vi "UniPend - ControlDesign.vi"() -> ()   [LabVIEW 2012]
uses:
  <vilib>/addons/Control Design/_Model Construction/Model Typedefs.llb/CD State Space Model (MIMO).ctl
  <vilib>/addons/Control Design/_Model Construction/Model Typedefs.llb/CD General Elements.ctl
  <vilib>/addons/Control Design/_Utility/Model Viewer.llb/Model Viewer SubVI/cd_Draw State-Space Equation (SS).vi
  <vilib>/addons/Control Design/_State Feedback Control/State Feedback Control.llb/State Feedback Control SubVis/cd_Discretized Linear Quadratic Regulator.vi
  <vilib>/addons/Control Design/_Model Conversions/Continuous and Discrete.llb/Continuous and Discrete SubVI/cd_Convert Continuous to Discrete (SS).vi
  <vilib>/addons/Control Design/_State Feedback Control/State Feedback Control.llb/CD State Regulator.vi
  <vilib>/addons/Control Design/_Model Reduction/Model Reduction.llb/Model Reduction SubVIs/cd_Remove I-O-S from SS Model.vi
  <vilib>/addons/Control Design/_Frequency Response Analysis/Frequency Response.llb/Frequency Response subVI/cd_Bode (State Space).vi
  <vilib>/addons/Control Design/_Time Response Analysis/Time Response.llb/Time Response subVI/cd_Impulse Response (State-Space).vi
  <vilib>/addons/Control Design/_Time Response Analysis/Time Response.llb/Time Response subVI/cd_Parametric Time Response (SS with External Response).vi
  <vilib>/addons/Control Design/_Dynamic Analysis/Dynamic Analysis.llb/Dynamic Analysis subVI/cd_Pole-Zero Map (State-Space).vi
  <vilib>/addons/Control Design/_Dynamic Analysis/Dynamic Analysis.llb/Dynamic Analysis subVI/cd_Stability (State-Space).vi
  <vilib>/addons/Control Design/_Model Conversions/NI_CD_Continuous and Discrete.lvlib
  <vilib>/addons/Control Design/_State Feedback Control/NI_CD_State Feedback Control.lvlib
  <vilib>/addons/Control Design/_Utility/NI_LinSys_Polynomial Math.lvlib
  <vilib>/addons/Control Design/_Utility/NI_CD_Model Viewer.lvlib
  <vilib>/addons/Control Design/_Model Reduction/NI_CD_Model Reduction.lvlib
  <vilib>/addons/Control Design/_Dynamic Analysis/NI_CD_Dynamic Analysis.lvlib
  <vilib>/addons/Control Design/_Time Response Analysis/NI_CD_Time Response.lvlib
  <vilib>/addons/Control Design/_Frequency Response Analysis/NI_CD_Frequency Response.lvlib
  <vilib>/addons/Control Design/_Model Construction/NI_LinSys_Model Typedefs.lvlib
panel:
  in  "Master Tab":T1(tab)
  out "Optimal Gain":dbl[](array[numeric])=[-16.081278889113918, -16.397482495141958, -3.1902773104017657, -2.0364914176335533] format="%.2f"
  in  "Tab Control":T2(tab)
  out "Linearized Equation for Operating Point":picture
  out "State-Space Model":T3={"properties"={"Model name"="", "Input names"=["Torque (Tau)"], "Output names"=["theta1", "theta2"], "Input Delays"=[0.0], "Output Delays"=[0.0, 0.0], "Sampling Time"=0.0, "Notes"=""}, "A"=[[0.0, 0.0, 1.0, 0.0], [0.0, 0.0, 0.0, 1.0], [-54.92473360770753, 40.408778283769514, -1.4920114239882594, 7.105427357601002e-15], [45.63201235945519, 58.19855210917706, 1.492011423988302, -0.22573956409963358]], "B"=[[0.0], [0.0], [29.84022847976503], [3.9334375679108007]], "C"=[[1.0, 0.0, 0.0, 0.0], [0.0, 0.9999999998433566, 0.0, 0.0]], "D"=[[0.0], [0.0]], "StateNames"=["/teta1", "/teta2", "/dteta1", "/dteta2"], "Transport Delay"=[[0.0], [0.0]]} {"Transport Delay" format="%.2f"; "D" format="%#.2g"; "C" format="%#.2g"; "B" format="%#.2g"; "A" format="%#.2g"; "properties"."Sampling Time" format="%#.6p"; "properties"."Output Delays" format="%.4f"; "properties"."Input Delays" format="%.4f"}
  in  "Control Technique":T5(tab)
  in  "Desired Pole Location":cdb[](array[numeric])=[0.8275428216771237+0.0i, 0.9068860314786581+0.0i, 0.9511525717602396+0.0i, 0.9425028249515996+0.0i] format="%.2f"
  in  "Q":dbl[][](array[numeric])=[[10.0, 0.0, 0.0, 0.0], [0.0, 10.0, 0.0, 0.0], [0.0, 0.0, 100.0, 0.0], [0.0, 0.0, 0.0, 1.0]] format="%.2f"
  in  "R":dbl[][](array[numeric])=[[50.0]] format="%.2f"
  in  "Acker Desired Pole Location":cdb[](array[numeric])=[0.8275428216771237+0.0i, 0.9068860314786581+0.0i, 0.9511525717602396+0.0i, 0.9425028249515996+0.0i] format="%.2f"
  out "Poles locations":cdb[](array[numeric])=[0.6612119646152013+0.0i, 0.9743397418352502+0.0i, 0.9379855295915182+0.0i, 0.9275584671894643+0.0i] format="%.2f"
  out "Gain":dbl[][](array[numeric])=[[13.362365480735772, 19.05380394095224, 1.2104119144158012, 2.4013527998190582]]
  out "Stability":T6(ring)
  out "Zeros":cdb[](array[numeric]) format="%.4f"
  out "Poles":cdb[](array[numeric])=[-30.459733943866535+0.0i, -2.5043848732190277+0.0i, -7.159085784207853+0.6196593444828095i, -7.159085784207853-0.6196593444828095i] format="%.4f"
  out "Pole-Zero Map":cluster{dbl[], dbl[]}[](graph)=[{[-30.459733943866535, -2.5043848732190277, -7.159085784207853, -7.159085784207853], [0.0, 0.0, 0.6196593444828095, -0.6196593444828095]}, {[], []}] caption="Closed Loop System Poles"
  out "Impulse Response":cluster{"time":dbl[], dbl[]}[](graph)
  out "Settling Time 1":dbl=2.363776391897807
  out "Settling Time 2":dbl=2.488531257025747
  out "Bode Magnitude":cluster{"W":dbl[], "Magnitude":dbl[]}[](graph)
  out "Bode Phase":cluster{"W":dbl[], "Magnitude":dbl[]}[](graph)
  in  "STOP Button":bool
  # "3-Phase 12 V Hub Motor"
  # "MicroStrain 3DM-GX3-45"
  # "RoboteQ Motor Controller"
  # "cRIO 9024 RT Controller"
  # "Unicycle Robot Design"
  # "IMU Sensor Reading"
  # "Control Technique"
  # "Hub Motor"
  # "System Controller Feedback Gain"
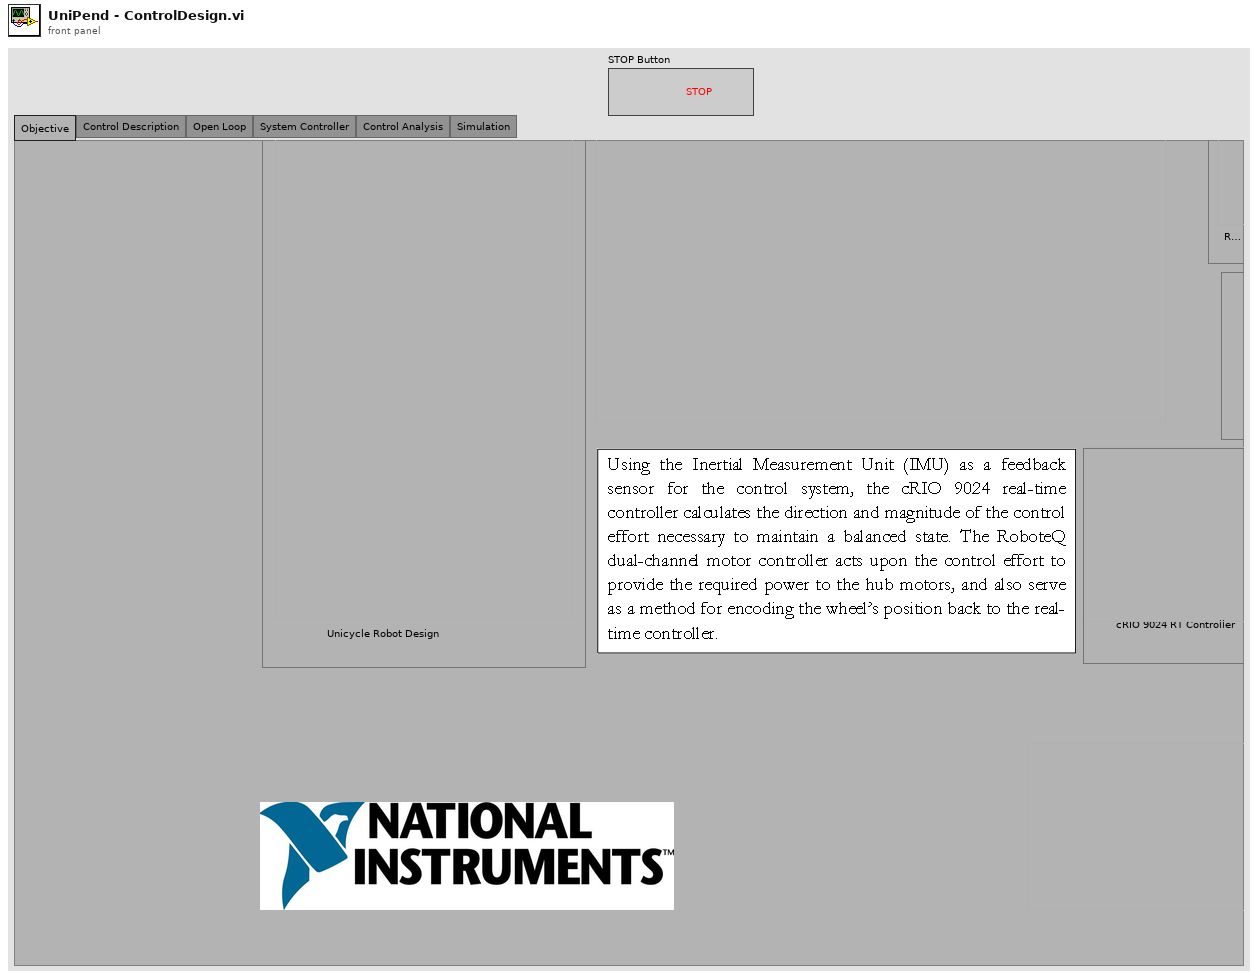
[diagram p1: front panel]
types:
  T1 = enum32{"Objective", "Control Description", "Open Loop", "System Controller", "Control Analysis", "Simulation"}
  T2 = enum32{"Discrete Model Info", "Discrete State Vector Info"}
  T3 = typedef "NI_LinSys_Model Typedefs.lvlib/CD State Space Model (MIMO).ctl" = cluster{"properties":T4, "A":dbl[][], "B":dbl[][], "C":dbl[][], "D":dbl[][], "StateNames":string[], "Transport Delay":dbl[][]}
  T4 = typedef "NI_LinSys_Model Typedefs.lvlib/CD General Elements.ctl" = cluster{"Model name":string, "Input names":string[], "Output names":string[], "Input Delays":dbl[], "Output Delays":dbl[], "Sampling Time":dbl, "Notes":string}
  T5 = enum32{"Pole Placement", "Linear Quadratic Regulator", "Ackermann"}
  T6 = enum16{"stable", "marginally stable", "unstable", "undetermined"}
  T7 = typedef "NI_LinSys_Data Typedefs.lvlib/CD MIMO Time Response Data.ctl" = cluster{"Time":dbl[], "Outputs Data":dbl[][][], "States Data":dbl[][][], "plot type":T8}
  T8 = typedef "NI_LinSys_Data Typedefs.lvlib/CD Plot Types Enum.ctl" = enum16{"bode-magnitude", "bode-phase", "nichols", "nyquist", "singular values", "step", "impulse", "initial", "simulation", "nyquist with separation"}
  T9 = typedef "NI_LinSys_Data Typedefs.lvlib/CD Parametric Time Response Data.ctl" = cluster{"Rise Time (s)":dbl[][], "Peak Time (s)":dbl[][], "Settling Time (s)":dbl[][], "Overshoot (%)":dbl[][], "Steady-State Gain":dbl[][], "Peak Value":dbl[][]}
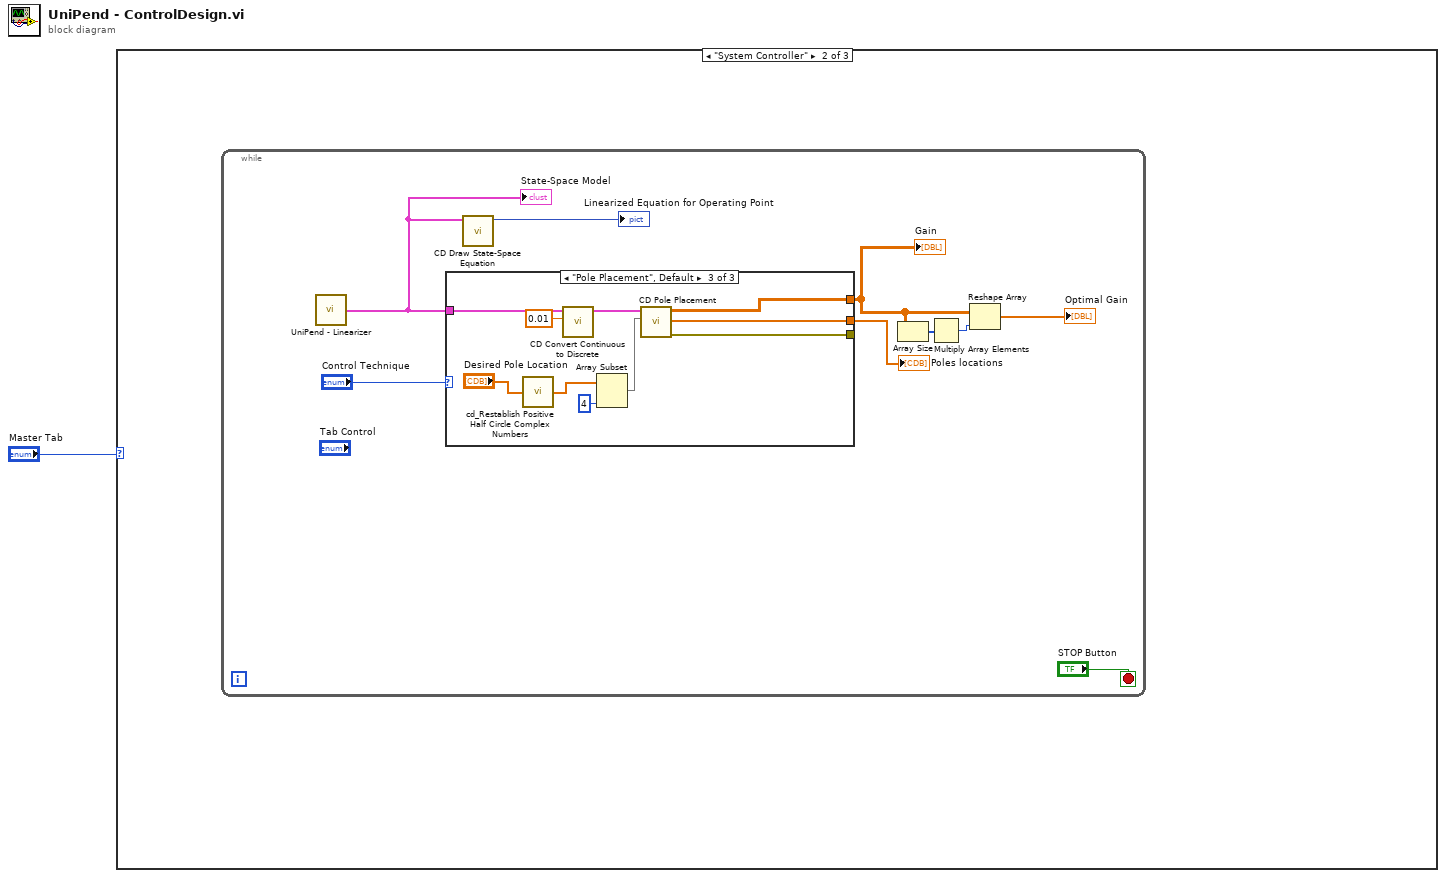
[diagram p0: block diagram]
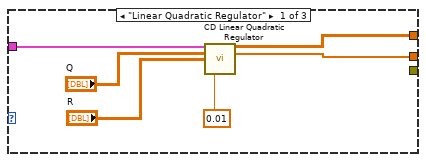
[diagram p3: hidden frame]
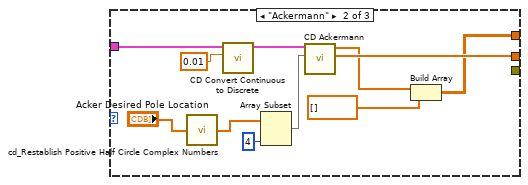
[diagram p4: hidden frame]
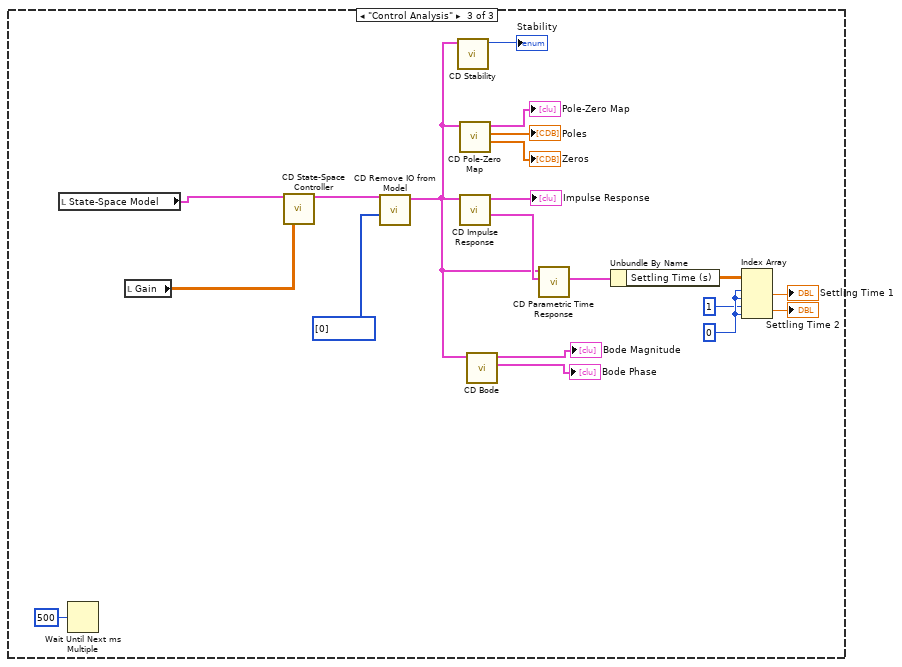
[diagram p5: hidden frame]
diagram:
  n1 = case shown="\"System Controller\"" "Master Tab" {
    frame "Objective", Default {
    }
    frame "System Controller" {
      n2 = while {
        stop <- "STOP Button" stop-if-true
        n3 = call "UniPend - Linearizer.vi"() -> ("State-Space Model"=w4:T3)  [unwired: 5 in]
        "State-Space Model" <- w4
        n4 = case shown="\"Pole Placement\", Default" "Control Technique" {
          tunnel: [w16 w17 w37] -> w5
          tunnel: w4 -> [w15 w22 w33]
          tunnel: [w12 w27 w36] -> w7
          tunnel: [_ _ w34] -> _
          frame "Linear Quadratic Regulator" {
            n5 = call-poly <vilib>:"CD Linear Quadratic Regulator.vi"("Continuous State-Space Model"=w15, "Q"="Q", "R"="R", "Sampling Time (s)"=0.01) -> ("Optimal Gain (K)"=w16:dbl[][], "Eigenvalues"=w12:cdb[])  [unwired: 2 in, 8 out]
          }
          frame "Ackermann" {
            n6 = call <vilib>:"cd_Restablish Positive Half Circle Complex Numbers.vi"("Sorted Complex Numbers (Positive Only)"="Acker Desired Pole Location") -> ("Complete Roots"=w25:cdb[])  [unwired: 8 out]
            n7 = call-poly <vilib>:"CD Convert Continuous to Discrete.vi"("Sampling Time (s)"=0.01, "Continuous State-Space Model"=w22) -> ("Discrete State-Space Model"=w21:T3)  [unwired: 7 in, 2 out]
            n8 = Array Subset(array=w25, length=4) -> (w20:cdb[])  [unwired: 1 in]
            n9 = call <vilib>:"CD Ackermann.vi"("Poles"=w20, "State-Space Model"=w21) -> ("Actual Poles"=w27:cdb[], "Gain"=w19:dbl[])  [unwired: 7 in, 1 out]
            n10 = Build Array(w19, dbl[] [] ("element")) -> (w17:dbl[][])
          }
          frame "Pole Placement", Default {
            n11 = call <vilib>:"cd_Restablish Positive Half Circle Complex Numbers.vi"("Sorted Complex Numbers (Positive Only)"="Desired Pole Location") -> ("Complete Roots"=w30:cdb[])  [unwired: 8 out]
            n12 = call-poly <vilib>:"CD Convert Continuous to Discrete.vi"("Sampling Time (s)"=0.01, "Continuous State-Space Model"=w33) -> ("Discrete State-Space Model"=w32:T3)  [unwired: 7 in, 2 out]
            n13 = Array Subset(array=w30, length=4) -> (w28:cdb[])  [unwired: 1 in]
            n14 = call <vilib>:"CD Pole Placement.vi"("Poles"=w28, "State-Space Model"=w32) -> ("error out"=w34:errorcluster, "Actual Poles"=w36:cdb[], "Gain"=w37:dbl[][])  [unwired: 2 in, 5 out]
          }
        }
        "Poles locations" <- w7
        "Gain" <- w5
        n15 = call-poly <vilib>:"CD Draw State-Space Equation.vi"("State-Space Model"=w4) -> ("Equation"=→"Linearized Equation for Operating Point":picture)  [unwired: 4 in, 6 out]
        n16 = Array Size(array=w5) -> (size(s)=w9:i32[])
        n17 = Multiply Array Elements(1:w9) -> (0:w8:i32)
        n18 = Reshape Array(w5, w8) -> (→"Optimal Gain":dbl[])
      }
    }
    frame "Control Analysis" {
      w45 = 0 ("index (row)")
      n19 = local read "State-Space Model"() -> (w57:T3)
      n20 = Wait Until Next ms Multiple(millisecond multiple=u32 500) -> ()  [unwired: 1 out]
      n21 = local read "Gain"() -> (w56:dbl[][])
      n22 = call-poly <vilib>:"CD State-Space Controller.vi"("State-Space Model"=w57, "Controller Gain (K)"=w56) -> ("Controller Model"=w54:T3)  [unwired: 12 in, 1 out]
      n23 = call-poly <vilib>:"CD Remove IO from Model.vi"("State-Space Model"=w54, "Outputs"=i32[] [0]) -> ("Reduced Model"=w40:T3)  [unwired: 7 in, 1 out]
      n24 = call-poly <vilib>:"CD Stability.vi"("State-Space Model"=w40) -> ("Stability"=→"Stability":T6)  [unwired: 8 in, 2 out]
      n25 = call-poly <vilib>:"CD Pole-Zero Map.vi"("State-Space Model"=w40) -> ("Zeros"=→"Zeros":cdb[], "Poles"=→"Poles":cdb[], "Pole-Zero Map"=→"Pole-Zero Map":cluster{dbl[], dbl[]}[])  [unwired: 7 in, 1 out]
      n26 = call-poly <vilib>:"CD Impulse Response.vi"("State-Space Model"=w40) -> ("Impulse Response Data"=w47:T7, "Impulse Response Graph"=→"Impulse Response":cluster{"time":dbl[], dbl[]}[])  [unwired: 7 in, 2 out]
      n27 = call-poly <vilib>:"CD Bode.vi"("State-Space Model"=w40) -> ("Bode Phase"=→"Bode Phase":cluster{"W":dbl[], "Magnitude":dbl[]}[], "Bode Magnitude"=→"Bode Magnitude":cluster{"W":dbl[], "Magnitude":dbl[]}[])  [unwired: 6 in, 3 out]
      n28 = call-poly <vilib>:"CD Parametric Time Response.vi"("Time Response Data"=w47, "State-Space Model"=w40) -> ("Time Response Parametric Data"=w41:T9)  [unwired: 8 in, 1 out]
      n29 = Unbundle By Name(w41) -> ("Settling Time (s)"=w42:dbl[][])
      n30 = Index Array(array=w42, index (row) #1=w45, index (col) #1=w45, index (row) #2=1 ("index (row)"), index (col) #2=w45) -> (element #1=→"Settling Time 1":dbl, element #2=→"Settling Time 2":dbl)
    }
  }
